vi "USBImageContinuousV1.8.vi"() -> ()   [LabVIEW 2019]
uses:
  atmcd32d.dll
panel:
  in  "Tab Control":T1(tab)
  out "Expected position on spectrometer (pixels):":dbl
  in  "Harmonic":dbl min=10.0 max=40.0
  out "l (nm)":dbl
  out "E (J)":dbl
  out "E (eV)":dbl
  out "Nearest Harmonic of 800nm":dbl
  out "Cursor Position (pixels)":dbl
  out "Distance to nearest harmonic of 800nm (pixels)":dbl
  in  "Grating:":u16(ring) items=["Shimadzu 30-006  "]
  in  "Laser:":u16(ring) items=["800nm  "]
  in  "Trigger":u32(ring) items=["Internal", "External"]
  in  "Exposure Time (secs)":sgl format="%.2f"
  out "Get Acquired Data":u32
  out "Start Acquisition":u32
  out "Detector X Pixels":i32
  out "Detector Y Pixels":i32
  out "Shut Down":u32
  out "Raw Image":i32[][](graph)
  out "Vertical Binned image":i32[](graph)
  out "Get Status":u32
  in  "Stop":bool
  in  "Save Image":bool
  out "Camera Status:":bool
  out "Last Image Saved:":string
  in  "Calibration Date":u16(ring) items=["first calibration - 7/31", "7/31-current"]
  out "Calibration Date: indicator:":u16(ring) items=["first calibration - 7/31", "7/31-current"]
  out "Status":u32
  out "Camera outputs":T2
  out "Camera inputs":T3
  in  "Correct for QE?":bool
  out "Wavelength Graph (nm)":T4(graph)
  out "Energy Graph (eV)":cluster{"eV":dbl, "QE scaled count":dbl}[](graph)
  out "Harmonics Graph":cluster{dbl, "QE scaled count":dbl}[](graph)
  # "Acquisition Mode: Single Scan\nReadout Mode: Full Resolution Image"
  # "Return values"
  # "XUV Spectrometer Control VI"
  # "Status"
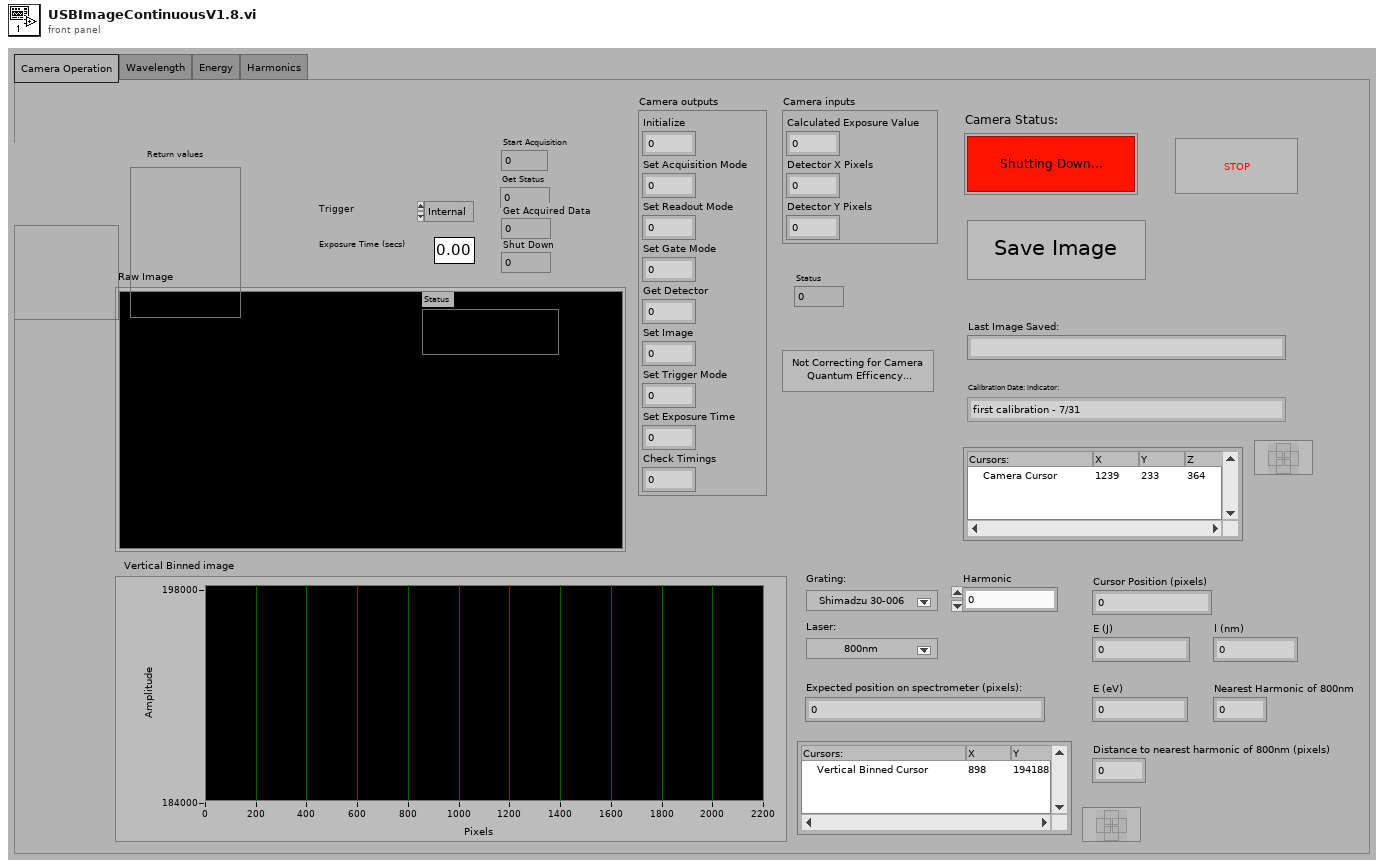
[diagram p1: front panel]
types:
  T1 = enum32{"Camera Operation", "Wavelength", "Energy", "Harmonics"}
  T2 = cluster{"Initialize":u32, "Set Acquisition Mode":u32, "Set Readout Mode":u32, "Set Gate Mode":u32, "Get Detector":u32, "Set Image":u32, "Set Trigger Mode":u32, "Set Exposure Time":u32, "Check Timings":u32}
  T3 = cluster{"Calculated Exposure Value":sgl, "Detector X Pixels":i32, "Detector Y Pixels":i32}
  T4 = cluster{"No prefix":dbl, "QE scaled count":dbl}[]
  T5 = cluster{"to shutdown":bool, "to get acquired data":bool, "to start acquisition":bool, "DRV_SUCCESS":i32}
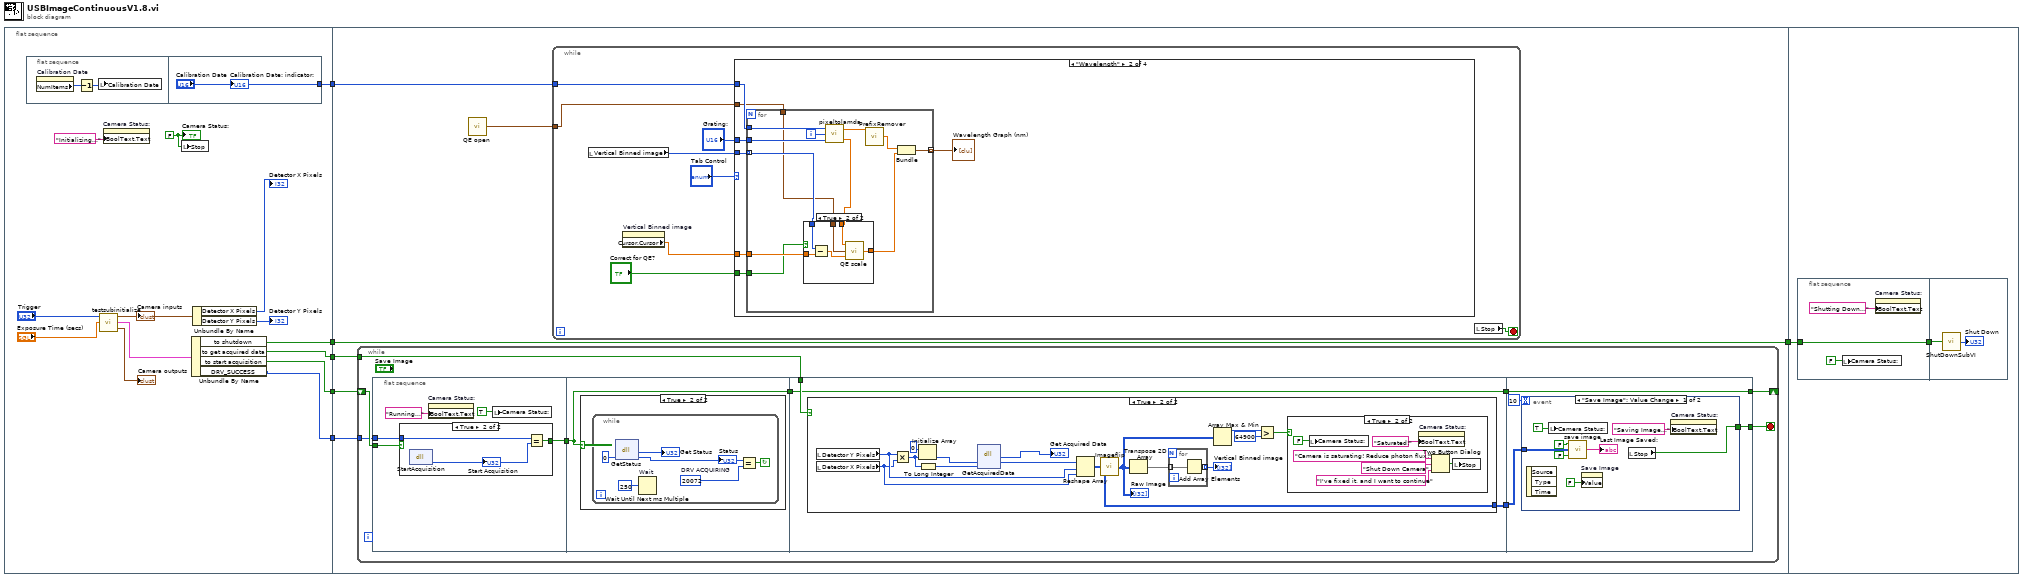
[diagram p0: block diagram]
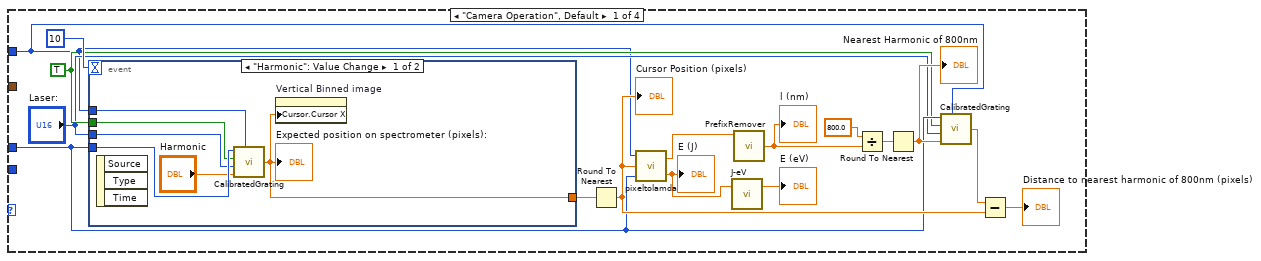
[diagram p2: hidden frame]
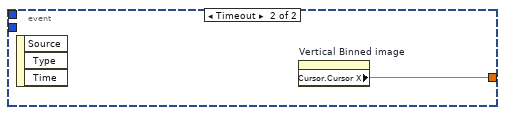
[diagram p3: hidden frame]
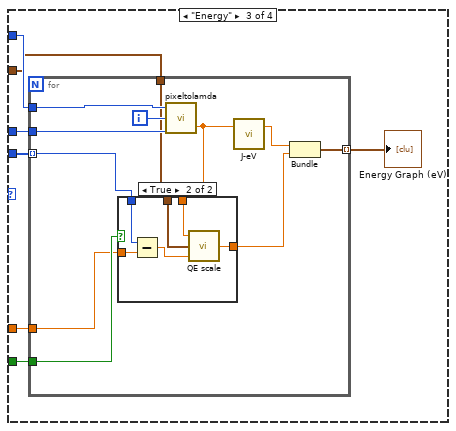
[diagram p5: hidden frame]
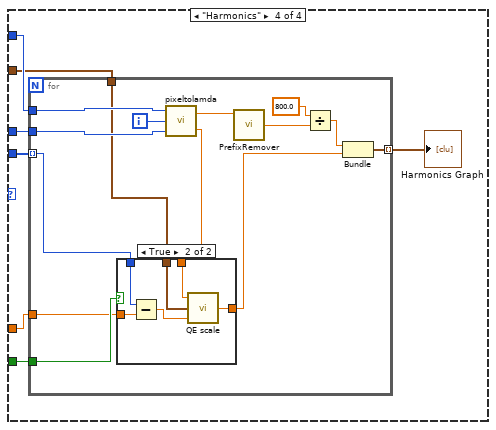
[diagram p7: hidden frame]
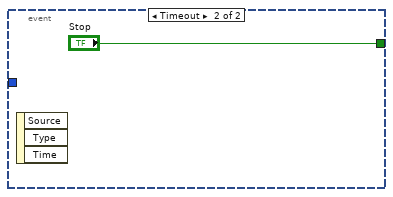
[diagram p13: hidden frame]
diagram:
  n1 = flat-sequence {
    tunnel: [w7] -> w5
    tunnel: [w8] -> w4
    tunnel: [w9] -> w3
    tunnel: [w10] -> w2
    tunnel: [w20] -> w1
    tunnel: [w26] -> w6
    tunnel: w5 -> [w29]
    tunnel: w4 -> [w28]
    tunnel: w3 -> [w27]
    tunnel: w2 -> [w26]
    tunnel: w1 -> [w25]
    tunnel: w6 -> [w204]
    frame #0 {
      w19 = FALSE ("Camera Status:")
      n2 = flat-sequence {
        tunnel: ["Calibration Date"] -> w20
        frame #0 {
          n3 = property on="Calibration Date" class="Ring (strict)"() -> ("NumItems"=w22:u32)  [unwired: 2 in, 2 out]
          n4 = Decrement(x=w22) -> (x-1=w21:u32)
          n5 = local write "Calibration Date"(w21) -> ()
        }
        frame #1 {
          "Calibration Date: indicator:" <- "Calibration Date"
        }
      }
      n6 = call "testsubinitialize.vi"("Exposure Time (secs)"="Exposure Time (secs)", "Trigger"="Trigger") -> ("Camera outputs"=→"Camera outputs":T2, "Camera status"=w17:T5, "Camera inputs"=w14:T3)  [unwired: 1 in]
      "Camera inputs" <- w14
      n7 = property on="Camera Status:" class="Bool (strict)"("BoolText.Text"="Initializing..." ("String")) -> ()  [unwired: 2 in, 2 out]
      n8 = local write "Stop"(w19) -> ()
      n9 = Unbundle By Name(w17) -> ("to shutdown"=w10:bool, "to get acquired data"=w9:bool, "to start acquisition"=w8:bool, "DRV_SUCCESS"=w7:i32)
      n10 = Unbundle By Name(w14) -> ("Detector X Pixels"=→"Detector X Pixels":i32, "Detector Y Pixels"=→"Detector Y Pixels":i32)
      "Camera Status:" <- w19
    }
    frame #1 {
      n11 = while {
        tunnel: w29 -> [w147]
        tunnel: w27 -> [w146]
        shift-right: [w142] -> _
        shift-left: w28 -> [w148]
        stop <- w140 stop-if-true
        n12 = flat-sequence {
          tunnel: w148 -> [w153]
          tunnel: w147 -> [w152]
          tunnel: [w151] -> w145
          tunnel: w145 -> [w158]
          tunnel: [w158] -> w144
          tunnel: w144 -> [w166]
          tunnel: w146 -> [w167]
          tunnel: [w166] -> w143
          tunnel: [w165] -> w141
          tunnel: w143 -> [w194]
          tunnel: w141 -> [w191]
          tunnel: [w192] -> w140
          tunnel: [w194] -> w142
          frame #0 {
            n13 = case shown="True" w153 {
              tunnel: [FALSE w157] -> w151
              tunnel: w152 -> [_ w156]
              frame False {
              }
              frame True {
                n14 = dll-call lib="atmcd32d.dll" fn="StartAcquisition" label="Call Library Function start acquisition"() -> (w155:u32)  [unwired: 3 in, 2 out]
                "Start Acquisition" <- w155
                n15 = Equal?(x=w156, y=w155) -> (x = y?=w157:bool)
              }
            }
            n16 = property on="Camera Status:" class="Bool (strict)"("BoolText.Text"="Running..." ("Boolean Text.Text")) -> ()  [unwired: 2 in, 2 out]
            n17 = local write "Camera Status:"(TRUE ("Camera Status:")) -> ()
          }
          frame #1 {
            n18 = case shown="True" w158 {
              frame False {
              }
              frame True {
                n19 = while {
                  stop <- w162 continue-if-true
                  w161 = u16 20072  # DRV ACQUIRING
                  n20 = dll-call lib="atmcd32d.dll" fn="GetStatus" label="Call Library Function GetAcquisitionStatus"(u16 0) -> (→"Get Status":u32, w160:u32)  [unwired: 3 in, 2 out]
                  "Status" <- w160
                  n21 = Wait Until Next ms Multiple "Wait"(millisecond multiple=u32 250) -> ()  [unwired: 1 out]
                  n22 = Equal?(x=w160, y=w161) -> (x = y?=w162:bool)
                }
              }
            }
          }
          frame #2 {
            n23 = case shown="True" w167 {
              tunnel: [_ w171] -> w165
              frame False {
              }
              frame True {
                n24 = local read "Detector Y Pixels"() -> (w177:i32)
                n25 = local read "Detector X Pixels"() -> (w173:i32)
                n26 = Multiply(x=w177, y=w173) -> (x*y=w179:i32)
                n27 = Initialize Array "Initialize Array"(0 ("Initial values in array"), w179) -> (w181:i32[])
                n28 = To Long Integer(number=w179) -> (32bit integer=w180:i32)
                n29 = dll-call lib="atmcd32d.dll" fn="GetAcquiredData" label="Call Library Function Get Acquired data"(w181, w180) -> (→"Get Acquired Data":u32, w178:i32[])  [unwired: 4 in, 2 out]
                n30 = Reshape Array(w178, w177, w173) -> (w171:i32[][])
                n31 = call "Imageflip.vi"("2D array"=w171) -> ("transposed array"=w169:i32[][])
                "Raw Image" <- w169
                n32 = Transpose 2D Array(2D array=w169) -> (transposed array=w176:i32[][])
                n33 = for {
                  tunnel: w176 -> [w190] mode=indexing
                  tunnel: [w189] -> w170 mode=indexing
                  n34 = Add Array Elements(numeric array=w190) -> (sum=w189:i32)
                }
                "Vertical Binned image" <- w170
                n35 = Array Max & Min(array=w169) -> (max value=w175:i32)  [unwired: 3 out]
                n36 = Greater?(x=w175, y=64900) -> (0:w174:bool)
                n37 = case shown="True" w174 {
                  frame False {
                  }
                  frame True {
                    n38 = local write "Camera Status:"(FALSE ("Camera Status:")) -> ()
                    n39 = property on="Camera Status:" class="Bool (strict)"("BoolText.Text"="Saturated!" ("Boolean Text.Text")) -> ()  [unwired: 2 in, 2 out]
                    n40 = Two Button Dialog(message="Camera is saturating! Reduce photon flux!", 1:"I've fixed it, and I want to continue" ("message"), 2:"Shut Down Camera" ("T button name (\"OK\")")) -> (T button?=w184:bool)
                    n41 = local write "Stop"(w184) -> ()
                  }
                }
              }
            }
          }
          frame #3 {
            n42 = event shown="[0] \"Save Image\": Value Change" {
              selector: _ -> [_ _]
              dyn-events: _ -> [_ _]
              timeout: 10 -> [_ _]
              tunnel: [w199 "Stop"] -> w192
              tunnel: w191 -> [w198 _]
              event "Save Image": Value Change {
                n43 = event-data() -> ()  [unwired: 1 in, 3 out]
                n44 = local write "Camera Status:"(TRUE ("Camera Status:")) -> ()
                n45 = call "save image.vi"("Start of pump/prove run?"=FALSE, "Image to save"=w198, "Pump/probe run?"=FALSE) -> ("Image file path"=→"Last Image Saved:":string)
                n46 = property on="Save Image" class="Bool (strict)"("Value"=FALSE ("Take image")) -> ()  [unwired: 2 in, 2 out]
                n47 = local read "Stop"() -> (w199:bool)
                n48 = property on="Camera Status:" class="Bool (strict)"("BoolText.Text"="Saving Image..." ("Boolean Text.Text")) -> ()  [unwired: 2 in, 2 out]
              }
              event Timeout {
                n49 = event-data() -> ()  [unwired: 1 in, 3 out]
              }
            }
          }
        }
      }
      n50 = call "QE open.vi"() -> ("QE data"=w24:cluster{"Numeric":dbl, dbl}[])
      n51 = while {
        tunnel: w25 -> [w33]
        tunnel: w24 -> [w32]
        stop <- w34 stop-if-true
        n52 = local read "Vertical Binned image"() -> (w36:i32[])
        n53 = property on="Vertical Binned image" class="WFGraph (strict)"() -> ("Cursor.Cursor Y"=w31:dbl)  [unwired: 2 in, 2 out]
        n54 = case shown="\"Wavelength\"" "Tab Control" {
          tunnel: w36 -> [_ w67 w93 w118]
          tunnel: "Grating:" -> [w41 w66 w92 w117]
          tunnel: w33 -> [w38 w64 w90 w115]
          tunnel: w32 -> [_ w63 w87 w114]
          tunnel: w31 -> [_ w62 w88 w112]
          tunnel: "Correct for QE?" -> [_ w61 w89 w113]
          frame "Camera Operation", Default {
            w40 = TRUE
            n55 = event shown="[0] \"Harmonic\": Value Change" {
              selector: _ -> [_ _]
              dyn-events: _ -> [_ _]
              timeout: 10 -> [_ _]
              tunnel: [w55 w60] -> w42
              tunnel: w41 -> [w59 _]
              tunnel: w40 -> [w58 _]
              tunnel: "Laser:" -> [w57 _]
              tunnel: w38 -> [w56 _]
              event "Harmonic": Value Change {
                n56 = event-data() -> ()  [unwired: 1 in, 3 out]
                n57 = call "CalibratedGrating.vi"("Grating:"=w59, "Subvi?"=w58, "Laser:"=w57, "Harmonic"="Harmonic", "Caibration Date"=w56) -> ("Position on spectrometer (pixels):"=w55:dbl)
                "Expected position on spectrometer (pixels):" <- w55
                n58 = property on="Vertical Binned image" class="WFGraph (strict)"("Cursor.Cursor X"=w55) -> ()  [unwired: 2 in, 2 out]
              }
              event Timeout {
                n59 = event-data() -> ()  [unwired: 1 in, 3 out]
                n60 = property on="Vertical Binned image" class="WFGraph (strict)"() -> ("Cursor.Cursor X"=w60:dbl)  [unwired: 2 in, 2 out]
              }
            }
            n61 = Round To Nearest(number=w42) -> (nearest integer value=w47:dbl)
            "Cursor Position (pixels)" <- w47
            n62 = call "pixeltolamda.vi"("Grating:"=w41, "Pixel Postion"=w47, "Caibration Date"=w38) -> ("E (J)"=w49:dbl, "lamda (m)"=w53:dbl)
            "E (J)" <- w49
            n63 = call "J-eV.vi"("J"=w49) -> ("eV"=→"E (eV)":dbl)  [unwired: 1 in, 1 out]
            n64 = call "PrefixRemover.vi"("Nano"=w53) -> ("No prefix"=w50:dbl)  [unwired: 3 in]
            "l (nm)" <- w50
            n65 = Divide(x=800.0, y=w50) -> (x/y=w52:dbl)
            n66 = Round To Nearest(number=w52) -> (nearest integer value=w46:dbl)
            "Nearest Harmonic of 800nm" <- w46
            n67 = call "CalibratedGrating.vi"("Grating:"=w41, "Subvi?"=w40, "Laser:"="Laser:", "Harmonic"=w46, "Caibration Date"=w38) -> ("Position on spectrometer (pixels):"=w45:dbl)
            n68 = Subtract(x=w45, y=w47) -> (x-y=→"Distance to nearest harmonic of 800nm (pixels)":dbl)
          }
          frame "Wavelength" {
            n69 = for {
              tunnel: w67 -> [w73] mode=indexing
              tunnel: w66 -> [w77]
              tunnel: [w75] -> w65 mode=indexing
              tunnel: w64 -> [w74]
              tunnel: w63 -> [w72]
              tunnel: w62 -> [w71]
              tunnel: w61 -> [w70]
              i -> [w76]
              n70 = call "pixeltolamda.vi"("Grating:"=w77, "Pixel Postion"=w76, "Caibration Date"=w74) -> ("E (J)"=w68:dbl, "lamda (m)"=w78:dbl)
              n71 = case shown="True" w70 {
                tunnel: w71 -> [_ w86]
                tunnel: w73 -> [w80 w85]
                tunnel: w72 -> [_ w83]
                tunnel: w68 -> [_ w82]
                tunnel: [w80 w81] -> w69
                frame False {
                }
                frame True {
                  n72 = Subtract(x=w85, y=w86) -> (x-y=w84:dbl)
                  n73 = call "QE scale.vi"("Raw Photon Count"=w84, "QE data"=w83, "Energy (J)"=w82) -> ("QE scaled count"=w81:dbl)
                }
              }
              n74 = call "PrefixRemover.vi"("Nano"=w78) -> ("No prefix"=w79:dbl)  [unwired: 3 in]
              n75 = Bundle("No prefix"=w79, "QE scaled count"=w69) -> (w75:cluster{"No prefix":dbl, "QE scaled count":dbl})  [unwired: 1 in]
            }
            "Wavelength Graph (nm)" <- w65
          }
          frame "Energy" {
            n76 = for {
              tunnel: w93 -> [w98] mode=indexing
              tunnel: w92 -> [w103]
              tunnel: [w101] -> w91 mode=indexing
              tunnel: w90 -> [w100]
              tunnel: w89 -> [w97]
              tunnel: w88 -> [w96]
              tunnel: w87 -> [w95]
              i -> [w104]
              n77 = call "pixeltolamda.vi"("Grating:"=w103, "Pixel Postion"=w104, "Caibration Date"=w100) -> ("E (J)"=w99:dbl)  [unwired: 1 out]
              n78 = case shown="True" w97 {
                tunnel: w96 -> [_ w111]
                tunnel: w98 -> [w105 w110]
                tunnel: w95 -> [_ w108]
                tunnel: w99 -> [_ w107]
                tunnel: [w105 w106] -> w94
                frame False {
                }
                frame True {
                  n79 = Subtract(x=w110, y=w111) -> (x-y=w109:dbl)
                  n80 = call "QE scale.vi"("Raw Photon Count"=w109, "QE data"=w108, "Energy (J)"=w107) -> ("QE scaled count"=w106:dbl)
                }
              }
              n81 = call "J-eV.vi"("J"=w99) -> ("eV"=w102:dbl)  [unwired: 1 in, 1 out]
              n82 = Bundle("eV"=w102, "QE scaled count"=w94) -> (w101:cluster{"eV":dbl, "QE scaled count":dbl})  [unwired: 1 in]
            }
            "Energy Graph (eV)" <- w91
          }
          frame "Harmonics" {
            n83 = for {
              tunnel: w118 -> [w122] mode=indexing
              tunnel: w117 -> [w131]
              tunnel: [w129] -> w116 mode=indexing
              tunnel: w115 -> [w125]
              tunnel: w114 -> [w124]
              tunnel: w113 -> [w120]
              tunnel: w112 -> [w119]
              i -> [w130]
              n84 = call "pixeltolamda.vi"("Grating:"=w131, "Pixel Postion"=w130, "Caibration Date"=w125) -> ("E (J)"=w123:dbl, "lamda (m)"=w132:dbl)
              n85 = case shown="True" w120 {
                tunnel: w119 -> [_ w139]
                tunnel: w122 -> [w133 w138]
                tunnel: w124 -> [_ w136]
                tunnel: w123 -> [_ w135]
                tunnel: [w133 w134] -> w121
                frame False {
                }
                frame True {
                  n86 = Subtract(x=w138, y=w139) -> (x-y=w137:dbl)
                  n87 = call "QE scale.vi"("Raw Photon Count"=w137, "QE data"=w136, "Energy (J)"=w135) -> ("QE scaled count"=w134:dbl)
                }
              }
              n88 = call "PrefixRemover.vi"("Nano"=w132) -> ("No prefix"=w127:dbl)  [unwired: 3 in]
              n89 = Divide(x=800.0, y=w127) -> (x/y=w126:dbl)
              n90 = Bundle(w126, "QE scaled count"=w121) -> (w129:cluster{dbl, "QE scaled count":dbl})  [unwired: 1 in]
            }
            "Harmonics Graph" <- w116
          }
        }
        n91 = local read "Stop"() -> (w34:bool)
      }
    }
    frame #2 {
      n92 = flat-sequence {
        tunnel: w204 -> [w208]
        tunnel: [w208] -> w205
        tunnel: w205 -> [w210]
        frame #0 {
          n93 = local write "Camera Status:"(FALSE ("Camera Status:")) -> ()
          n94 = property on="Camera Status:" class="Bool (strict)"("BoolText.Text"="Shutting Down..." ("Boolean Text.Text")) -> ()  [unwired: 2 in, 2 out]
        }
        frame #1 {
          n95 = call "ShutDownSubVI.vi"("shutdown"=w210) -> ("Shut Down"=→"Shut Down":u32)
        }
      }
    }
  }
